vi "FeedbackDecode_UDPStr2Single.vi"(1 "UDPStr":string) -> (0 "UDPSingle":sgl[](array[numeric]))   [LabVIEW 2020]
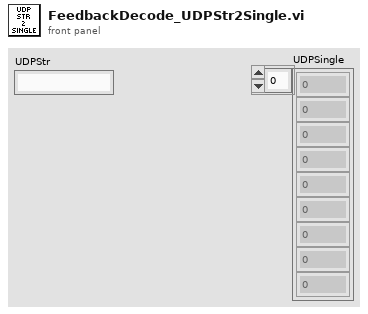
[diagram p1: front panel]
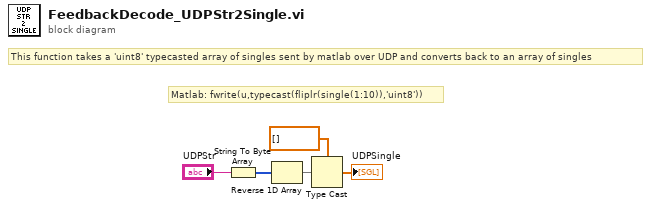
[diagram p0: block diagram]
diagram:
  # "This function takes a 'uint8' typecasted array of singles sent by matlab over UDP and converts back to an array of singles"
  # "Matlab: fwrite(u,typecast(fliplr(single(1:10)),'uint8'))"
  n1 = String To Byte Array(string="UDPStr") -> (unsigned byte array=w3:u8[])
  n2 = Reverse 1D Array(array=w3) -> (reversed array=w2:u8[])
  n3 = Type Cast(type=sgl[] [], x=w2) -> (*(type *) &x=→"UDPSingle":sgl[])
